vi "SERIAL_Open.vi"(7 "Serial Port (MXP)":T1=enum."MXP TTL", 10 "Update Rate (4Hz-60Hz)":u8=50, 11 "Nav6Mode (YPR)":T2) -> (0 "error out":errorcluster, 1 "Opened":bool, 3 "navX Ref":T3={"SerialPortRef"={"DevStatus"={"status"=FALSE, "code"=0, "source"=""}, "Serial Port Name"=""}, "Board Information"={"WhoAmI (50 | 0x32)"=0, "Board Revision"=0, "Firmware Major Version"=0, "Firmware Minor Version"=0}, "Status"={"Update Rate Hz"=0, "Accelerometer Full-Scale Range"=0, "Gyro Full-Scale Range"=0, "NAVX_OP_STATUS"=0, "NAVX_CAL_STATUS"=0, "NAVX_SELFTEST_STATUS"=0, "NAVX_SENSOR_STATUS"={"MOVING"=FALSE, "YAW_STABLE"=FALSE, "MAG_DISTURBANCE"=FALSE, "ALTITUDE_VALID"=FALSE, "SEALEVEL_PRESS_SET"=FALSE, "FUSED_HEADING_VALID"=FALSE}}, "Offsets"={"Yaw"=0.0, "Quat W"=0.0, "Quat X"=0.0, "Quat Y"=0.0, "Quat Z"=0.0}, "Update Rate (4Hz-60Hz)"=50, "Nav6Mode (YPR)"=enum."YPR", "refnum name"="", "error"={"status"=FALSE, "code"=0, "source"=""}} {"Status"."NAVX_OP_STATUS" items=["INITIALIZING", "SELFTEST_IN_PROGRESS", "ERROR", "IMU_AUTOCAL_IN_PROGRESS", "NORMAL"]; "Status"."NAVX_CAL_STATUS" items=["IMU_CAL_STATE_MASK"=3, "IMU_CAL_INPROGRESS"=0, "IMU_CAL_ACCUMULATE"=1, "IMU_CAL_COMPLETE"=2, "MAG_CAL_COMPLETE"=4, "BARO_CAL_COMPLETE"=8]})   [LabVIEW 2014, in "navX-MXP IMU.lvlib"]
uses:
  navX-MXP IMU.lvlib
  <vilib>/Rock Robotics/WPI/SerialPort/WPI_SerialPortRef.ctl
  Internal/navX Serial DevRef.ctl
  COMMON/TypeDefs/navX NAVX_CAL_STATUS.ctl
  COMMON/TypeDefs/navX NAVX_OP_STATUS.ctl
  COMMON/TypeDefs/navX Status Data.ctl
  COMMON/TypeDefs/navX Board Information.ctl
  TypeDefs/navX Serial Mode.ctl
  COMMON/TypeDefs/navX NAVX_SENSOR_STATUS.ctl
  NI WPI/WPI_SerialPort_USB.ctl
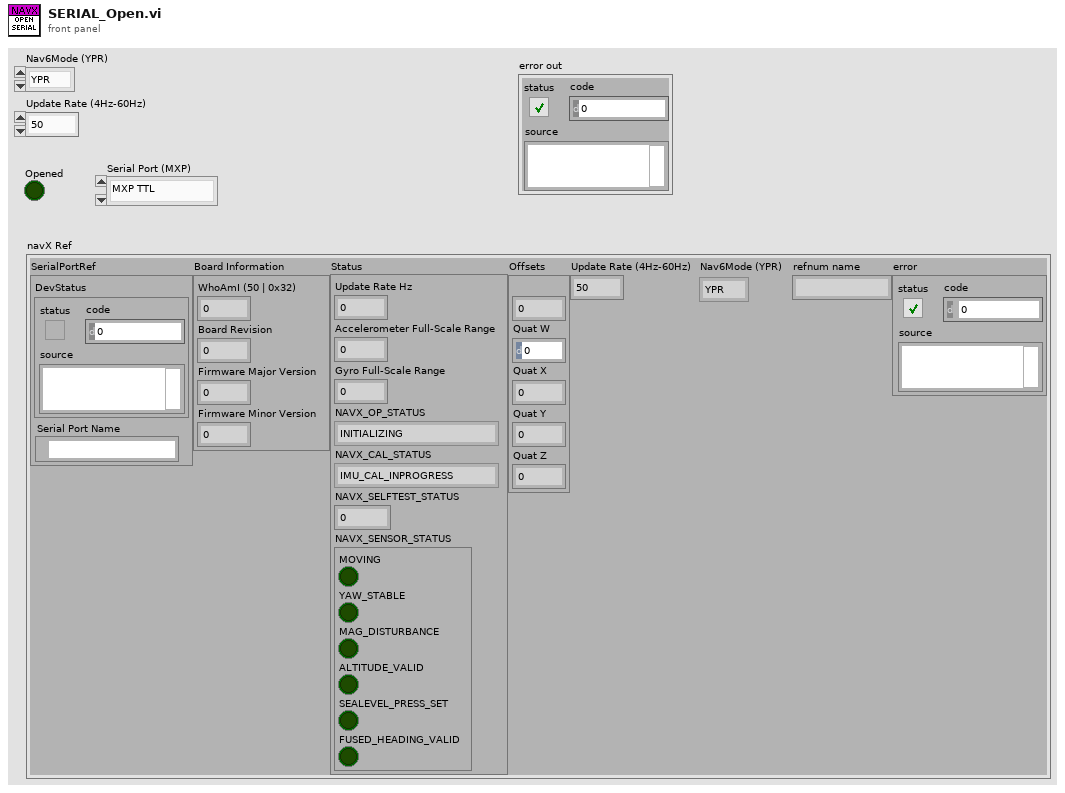
[diagram p1: front panel]
types:
  T1 = typedef "navX-MXP IMU.lvlib/WPI_SerialPort_USB.ctl" = enum16{"Onboard RS-232", "MXP TTL", "USB"}
  T2 = typedef "navX-MXP IMU.lvlib/navX Serial Mode.ctl" = enum16{"YPR", "Gyro", "Quaternion"}
  T3 = typedef "navX-MXP IMU.lvlib/navX Serial DevRef.ctl" = cluster{"SerialPortRef":T4, "Board Information":T5, "Status":T6, "Offsets":cluster{"Yaw":dbl, "Quat W":dbl, "Quat X":dbl, "Quat Y":dbl, "Quat Z":dbl}, "Update Rate (4Hz-60Hz)":u8, "Nav6Mode (YPR)":T2, "refnum name":string, "error":errorcluster}
  T4 = typedef "WPI_SerialPortRef.ctl" = cluster{"DevStatus":errorcluster, "Serial Port Name":refnum<visa-resource-name>}
  T5 = typedef "navX-MXP IMU.lvlib/navX Board Information.ctl" = cluster{"WhoAmI (50 | 0x32)":u8, "Board Revision":u8, "Firmware Major Version":u8, "Firmware Minor Version":u8}
  T6 = typedef "navX-MXP IMU.lvlib/navX Status Data.ctl" = cluster{"Update Rate Hz":u8, "Accelerometer Full-Scale Range":u8, "Gyro Full-Scale Range":u16, "NAVX_OP_STATUS":T7, "NAVX_CAL_STATUS":T8, "NAVX_SELFTEST_STATUS":u8, "NAVX_SENSOR_STATUS":T9}
  T7 = typedef "navX-MXP IMU.lvlib/navX NAVX_OP_STATUS.ctl" = u8
  T8 = typedef "navX-MXP IMU.lvlib/navX NAVX_CAL_STATUS.ctl" = u8
  T9 = typedef "navX-MXP IMU.lvlib/navX NAVX_SENSOR_STATUS.ctl" = cluster{"MOVING":bool, "YAW_STABLE":bool, "MAG_DISTURBANCE":bool, "ALTITUDE_VALID":bool, "SEALEVEL_PRESS_SET":bool, "FUSED_HEADING_VALID":bool}
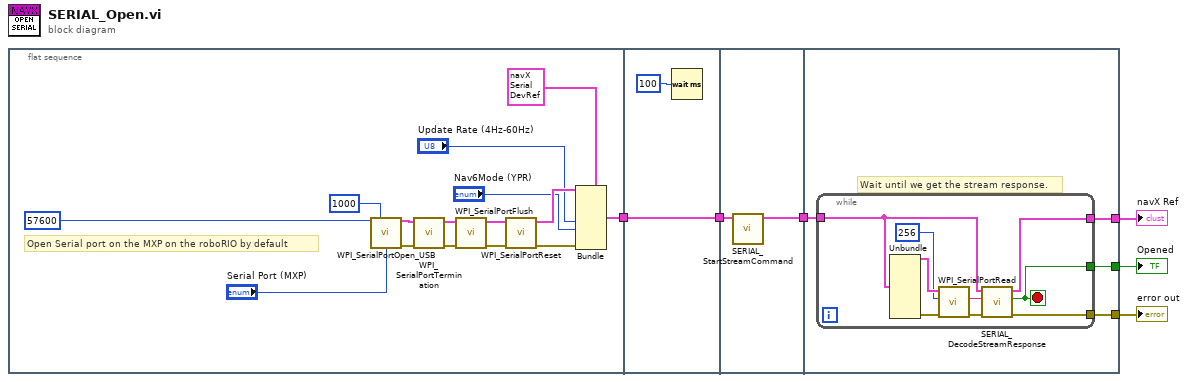
[diagram p0: block diagram]
diagram:
  n1 = flat-sequence {
    tunnel: [w11] -> w6
    tunnel: w6 -> [w23]
    tunnel: [w23] -> w5
    tunnel: w5 -> [w25]
    tunnel: [w24] -> w4
    tunnel: w4 -> [w27]
    tunnel: [w29] -> w1
    tunnel: [w28] -> w3
    tunnel: [w26] -> w2
    frame #0 {
      # "Open Serial port on the MXP on the roboRIO by default"
      n2 = call "WPI_SerialPortOpen_USB.vi"("Baud Rate"=u32 57600, "Timeout Value (ms)"=u32 1000, "Serial Port"="Serial Port (MXP)") -> ("SerialPortRef"=w18:T4, "error out"=w19:errorcluster)  [unwired: 11 in]
      n3 = call <vilib>:"WPI_SerialPortTermination.vi"("error in (no error)"=w19, "SerialPortRef"=w18) -> ("error out"=w17:errorcluster, "SerialPortRef"=w16:T4)  [unwired: 8 in]
      n4 = call <vilib>:"WPI_SerialPortFlush.vi"("error in (no error)"=w17, "SerialPortRef"=w16) -> ("error out"=w15:errorcluster, "SerialPortRef"=w14:T4)  [unwired: 8 in]
      n5 = call <vilib>:"WPI_SerialPortReset.vi"("error in (no error)"=w15, "SerialPortRef"=w14) -> ("error out"=w7:errorcluster, "SerialPortRef"=w12:T4)  [unwired: 8 in]
      n6 = Bundle(cluster=T3 {"SerialPortRef"={"DevStatus"={"status"=FALSE, "code"=0, "source"=""}, "Serial Port Name"=""}, "Board Information"={"WhoAmI (50 | 0x32)"=0, "Board Revision"=0, "Firmware Major Version"=0, "Firmware Minor Version"=0}, "Status"={"Update Rate Hz"=0, "Accelerometer Full-Scale Range"=0, "Gyro Full-Scale Range"=0, "NAVX_OP_STATUS"=0, "NAVX_CAL_STATUS"=0, "NAVX_SELFTEST_STATUS"=0, "NAVX_SENSOR_STATUS"={"MOVING"=FALSE, "YAW_STABLE"=FALSE, "MAG_DISTURBANCE"=FALSE, "ALTITUDE_VALID"=FALSE, "SEALEVEL_PRESS_SET"=FALSE, "FUSED_HEADING_VALID"=FALSE}}, "Offsets"={"Yaw"=0.0, "Quat W"=0.0, "Quat X"=0.0, "Quat Y"=0.0, "Quat Z"=0.0}, "Update Rate (4Hz-60Hz)"=50, "Nav6Mode (YPR)"=enum."YPR", "refnum name"="", "error"={"status"=FALSE, "code"=0, "source"=""}} ("navX Ref Object"), "SerialPortRef"=w12, "Update Rate (4Hz-60Hz)"="Update Rate (4Hz-60Hz)", "Nav6Mode (YPR)"="Nav6Mode (YPR)", "error"=w7) -> (w11:T3)  [unwired: 4 in]
    }
    frame #1 {
      n7 = Wait (ms)(milliseconds to wait=u32 100) -> ()  [unwired: 1 out]
    }
    frame #2 {
      n8 = call "SERIAL_StartStreamCommand.vi"("navX Ref"=w25) -> ("navX Ref"=w24:T3)  [unwired: 10 in]
    }
    frame #3 {
      # "Wait until we get the stream response."
      n9 = while {
        tunnel: [w35] -> w29
        tunnel: [w34] -> w28
        tunnel: w27 -> [w32]
        tunnel: [w30] -> w26
        stop <- w30 stop-if-true
        n10 = Unbundle(w32) -> ("SerialPortRef"=w38:T4, "error"=w33:errorcluster)  [unwired: 6 out]
        n11 = call <vilib>:"WPI_SerialPortRead.vi"("error in (no error)"=w33, "Num Bytes to Read"=u32 256, "SerialPortRef"=w38) -> ("error out"=w36:errorcluster, "Buffer"=w31:string)  [unwired: 6 in, 1 out]
        n12 = call "SERIAL_DecodeStreamResponse.vi"("error in"=w36, "Buffer"=w31, "navX DevRef"=w32) -> ("error out"=w34:errorcluster, "Valid"=w30:bool, "navX DevRef"=w35:T3)  [unwired: 6 in]
      }
    }
  }
  "error out" <- w3
  "navX Ref" <- w1
  "Opened" <- w2
